vi "SubVI ausfuehren.vi"(8 "Fehler":errorcluster caption="Fehler (Eingang, kein Fehler)", 10 "Referenz":refnum<vi>) -> (3 "vi reference":refnum<vi>)   [LabVIEW 2020, in "allgemeine Sub-VIs.lvlib"]
uses:
  allgemeine Sub-VIs.lvlib
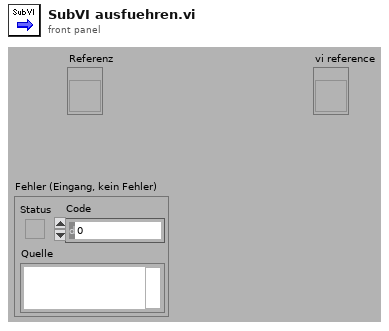
[diagram p1: front panel]
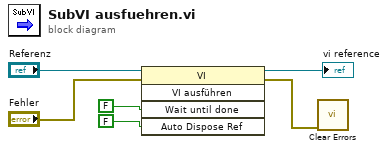
[diagram p0: block diagram]
diagram:
  n1 = invoke class="VI" method="VI ausführen"(reference="Referenz", error in="Fehler", "Wait until done"=FALSE ("Warten bis beendet"), "Auto Dispose Ref"=FALSE ("Referenz automatisch schließen")) -> (reference out=→"vi reference":refnum<vi>, error out=w1:errorcluster)  [unwired: 1 in, 3 out]
  n2 = call <vilib>:"Clear Errors.vi"("error in (no error)"=w1) -> ()  [unwired: 5 in, 2 out]
